vi "Read Measurement (Setup and Hold Time).vi"(0 "VISA resource name":refnum<visa-resource-name>, 1 "Data Source Direction (0: Rising)":i32(ring) items=["Rising", "Falling", "Both"], 2 "Clock Source (2: Channel 2)":i32(ring)=2 caption="Channel (1: Channel 1)" items=["Channel 1"=1, "Channel 2"=2, "Channel 3"=3, "Channel 4"=4, "Function 1"=5, "Function 2"=6, "Function 3"=7, "Function 4"=8, "Memory 1"=9, "Memory 2"=10, "Memory 3"=11, "Memory 4"=12, "Clock"=15, "MTrend"=16, "MSpectrum"=17, "Equalized"=18, "DIG 0"=20, "DIG 1"=21, "DIG 2"=22, "DIG 3"=23, "DIG 4"=24, "DIG 5"=25, "DIG 6"=26, "DIG 7"=27, "DIG 8"=28, "DIG 9"=29, "DIG 10"=30, "DIG 11"=31, "DIG 12"=32, "DIG 13"=33, "DIG 14"=34, "DIG 15"=35], 3 "Clock Source Direction (0: Rising)":i32(ring) items=["Rising", "Falling", "Both"], 5 "Data Source (1: Channel 1)":i32(ring)=1 caption="Channel (1: Channel 1)" items=["Channel 1"=1, "Channel 2"=2, "Channel 3"=3, "Channel 4"=4, "Function 1"=5, "Function 2"=6, "Function 3"=7, "Function 4"=8, "Memory 1"=9, "Memory 2"=10, "Memory 3"=11, "Memory 4"=12, "Clock"=15, "MTrend"=16, "MSpectrum"=17, "Equalized"=18], 7 "Measurement Function (0: Setup Time)":i32(ring) items=["Setup Time", "Hold Time"], 9 "Maximum Time (10000ms)":u32=10000, 11 "error in (no error)":errorcluster) -> (4 "VISA resource name out":refnum<visa-resource-name>, 6 "Setup or Hold Time (s)":dbl, 15 "error out":errorcluster)   [LabVIEW 2013, in "Agilent 90000 Series.lvlib"]
doc: "Measures the setup or hold time between the specified clock and data source.\n\nThis VI initiates an acquisition on the channel that the end-user defines. It then waits for the acquisition to complete, obtains a waveform measurement on the channel the end-user specifies, and returns the measurement value."
uses:
  Agilent 90000 Series.lvlib
  Low Level/Fetch Measurement (Setup and Hold Time).vi
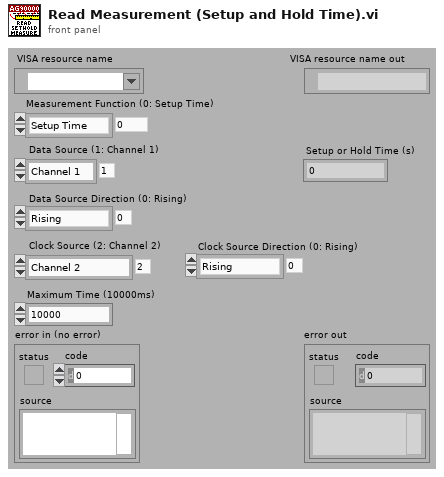
[diagram p1: front panel]
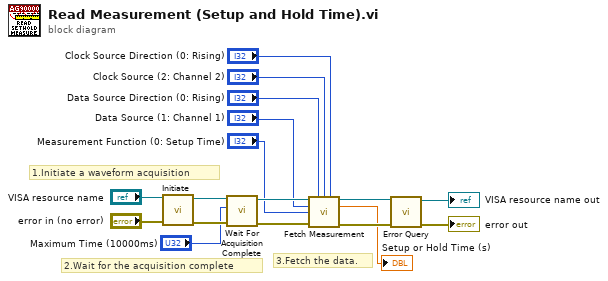
[diagram p0: block diagram]
diagram:
  # "3.Fetch the data."
  # "2.Wait for the acquisition complete"
  # "1.Initiate a waveform acquisition"
  n1 = call "Initiate.vi"("error in (no error)"="error in (no error)", "VISA resource name"="VISA resource name") -> ("error out"=w11:errorcluster, "VISA resource name out"=w10:refnum<visa-resource-name>)  [unwired: 8 out]
  n2 = call "Wait For Acquisition Complete.vi"("error in (no error)"=w11, "Maximum Time (10000ms)"="Maximum Time (10000ms)", "VISA resource name"=w10) -> ("error out"=w15:errorcluster, "VISA resource name out"=w14:refnum<visa-resource-name>)  [unwired: 7 out]
  n3 = call-poly "Fetch Measurement.vi"("VISA resource name"=w14, "Data Source Direction (0: Rising)"="Data Source Direction (0: Rising)", "Clock Source (2: Channel 2)"="Clock Source (2: Channel 2)", "Clock Source Direction (0: Rising)"="Clock Source Direction (0: Rising)", "Data Source (1: Channel 1)"="Data Source (1: Channel 1)", "Measurement Function (0: Setup Time)"="Measurement Function (0: Setup Time)", "error in (no error)"=w15) -> ("VISA resource name out"=w9:refnum<visa-resource-name>, "Setup or Hold Time (s)"=→"Setup or Hold Time (s)":dbl, "error out"=w8:errorcluster)  [unwired: 1 in, 5 out]
  n4 = call "Error Query.vi"("error in (no error)"=w8, "VISA resource name"=w9) -> ("error out"=→"error out":errorcluster, "VISA resource name out"=→"VISA resource name out":refnum<visa-resource-name>)  [unwired: 8 out]
